vi "OAT Single Stage Interpolation with IC.vi"(6 "initial state":dbl[](array[numeric]) format="%.2f", 8 "error in (no error)":errorcluster, 9 "filter":T1={"coefficients"=[], "factor"=1} {"coefficients" format="%.2f"}, 11 "X":dbl[](array[numeric]) format="%.2f") -> (0 "error out":errorcluster, 3 "Y":dbl[](array[numeric]) format="%.2f", 4 "final state":dbl[](array[numeric]) format="%.2f")   [LabVIEW 2017, in "SoundVib_Resampling.lvlib"]
doc: "Interpolate the input sequence <B>X</B> with the single stage interpolation filter specified by <B>filter</B>."
uses:
  <vilib>/addons/Sound and Vibration/Order Analysis/Resample Order Tracking/SoundVib_Resampling.lvlib
  <vilib>/addons/_NISVFA/_Shared subVIs/Controls/OAT Decimation Filter.ctl
  <resource>/sndvib.dll
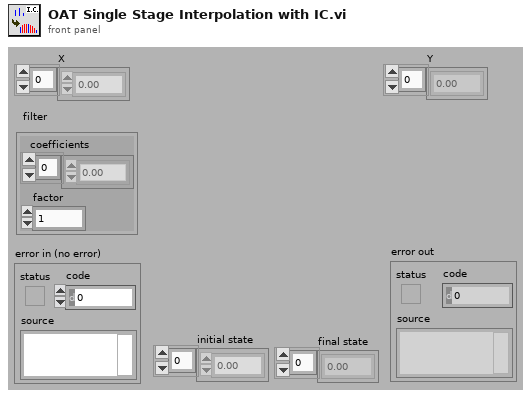
[diagram p1: front panel]
types:
  T1 = typedef "OAT Decimation Filter.ctl" = cluster{"coefficients":dbl[], "factor":i32}
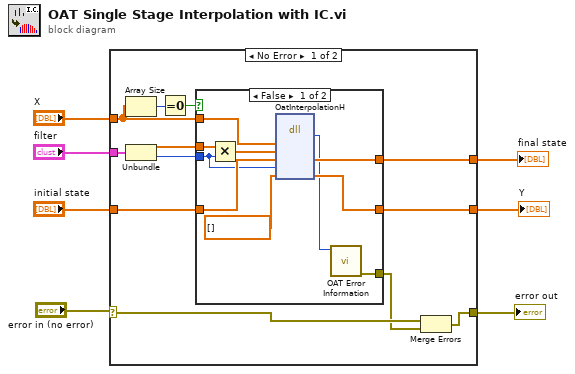
[diagram p0: block diagram]
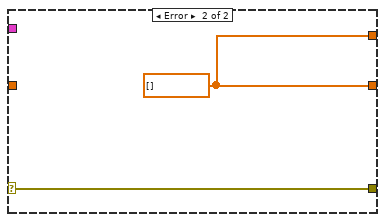
[diagram p3: hidden frame]
diagram:
  n1 = case shown="No Error" "error in (no error)" {
    selector: "error in (no error)" -> [w10 w33]
    tunnel: "initial state" -> [w19 _]
    tunnel: "filter" -> [w18 _]
    tunnel: "X" -> [w13 _]
    tunnel: [w17 w32] -> w4
    tunnel: [w16 w32] -> w3
    tunnel: [w8 w33] -> w1
    frame No Error {
      n2 = Array Size(array=w13) -> (size(s)=w12:i32)
      n3 = Unbundle(w18) -> ("coefficients"=w15:dbl[], "factor"=w14:i32)
      n4 = Equal To 0?(x=w12) -> (x = 0?=w11:bool)
      n5 = case shown="False" w11 {
        tunnel: w19 -> [w29 w31]
        tunnel: w13 -> [w28 w30]
        tunnel: [w27 w31] -> w17
        tunnel: [w26 w30] -> w16
        tunnel: w15 -> [w24 _]
        tunnel: w14 -> [w23 _]
        tunnel: [w20 _] -> w9
        frame False {
          n6 = Multiply(x=w24, y=w23) -> (x*y=w25:dbl[])
          n7 = dll-call lib="C:/Program Files (x86)/National Instruments/LabVIEW 2017/resource/sndvib.*" fn="OatInterpolationH"("xH"=w28, "filterH"=w25, "initH"=w29, "dec_factor"=w23, "yH"=dbl[] []) -> ("return type"=w21:i32, "initH"=w27:dbl[], "yH"=w26:dbl[])  [unwired: 6 in, 2 out]
          n8 = call <vilib>:"OAT Error Information.vi"("error code"=w21) -> ("error out"=w20:errorcluster)  [unwired: 6 in]
        }
        frame True {
        }
      }
      n9 = Merge Errors(w10, w9) -> (w8:errorcluster)
    }
    frame Error {
      w32 = dbl[] [] ("yH")
    }
  }
  "Y" <- w3
  "final state" <- w4
  "error out" <- w1
